vi "Path Flatness SLM.vi"() -> (8 "flatness path":path)   [LabVIEW 2014]
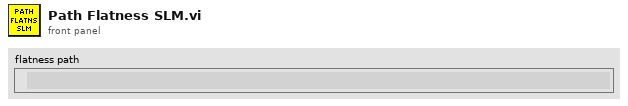
[diagram p1: front panel]
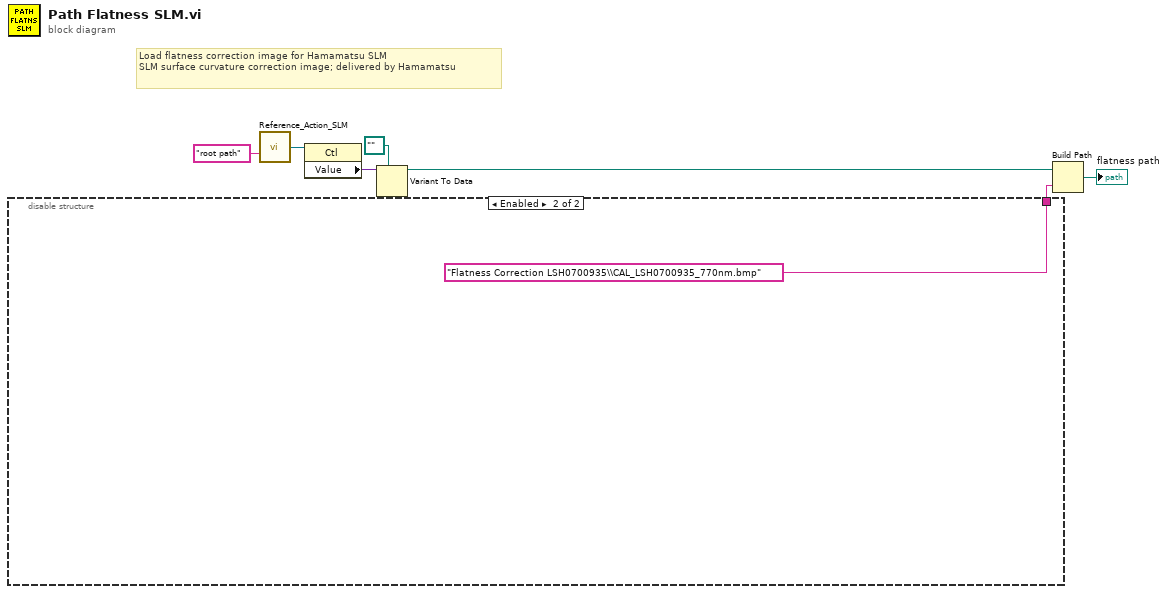
[diagram p0: block diagram]
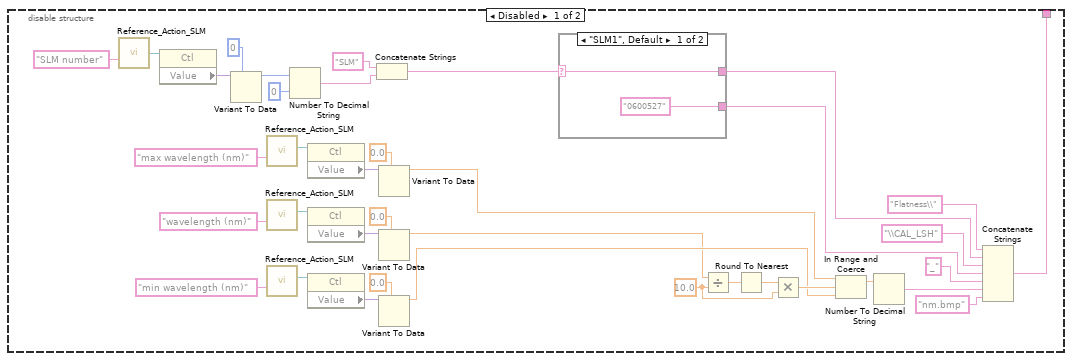
[diagram p2: hidden frame]
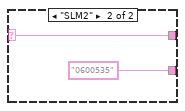
[diagram p3: hidden frame]
diagram:
  # "Load flatness correction image for Hamamatsu SLM\nSLM surface curvature correction image; delivered by Hamamatsu"
  n1 = disable-structure shown="Enabled" {
    disable-tunnel: [w17 "Flatness Correction LSH0700935\\CAL_LSH0700935_770nm.bmp"] -> w2
    frame Disabled {
      w24 = 10.0 ("y")
      n2 = call "Reference_Action_SLM.vi"("Control Name"="SLM number") -> ("Ref OUT"=w13:refnum<vi>)  [unwired: 12 in, 2 out]
      n3 = property class="Ctl"(reference=w13) -> ("Value"=w14:variant)  [unwired: 1 in, 2 out]
      n4 = Variant To Data(type=0, Variant=w14) -> (data=w10:i32)  [unwired: 1 in, 1 out]
      n5 = call "Reference_Action_SLM.vi"("Control Name"="max wavelength (nm)") -> ("Ref OUT"=w43:refnum<vi>)  [unwired: 12 in, 2 out]
      n6 = call "Reference_Action_SLM.vi"("Control Name"="wavelength (nm)") -> ("Ref OUT"=w39:refnum<vi>)  [unwired: 12 in, 2 out]
      n7 = call "Reference_Action_SLM.vi"("Control Name"="min wavelength (nm)") -> ("Ref OUT"=w35:refnum<vi>)  [unwired: 12 in, 2 out]
      n8 = Number To Decimal String(number=w10, width (-)=i16 0) -> (decimal integer string=w8:string)
      n9 = property class="Ctl"(reference=w43) -> ("Value"=w44:variant)  [unwired: 1 in, 2 out]
      n10 = property class="Ctl"(reference=w39) -> ("Value"=w40:variant)  [unwired: 1 in, 2 out]
      n11 = property class="Ctl"(reference=w35) -> ("Value"=w36:variant)  [unwired: 1 in, 2 out]
      n12 = Concatenate Strings("SLM" ("name or relative path"), w8) -> (w15:string)
      n13 = Variant To Data(type=0.0, Variant=w44) -> (data=w20:dbl)  [unwired: 1 in, 1 out]
      n14 = Variant To Data(type=0.0, Variant=w40) -> (data=w21:dbl)  [unwired: 1 in, 1 out]
      n15 = Variant To Data(type=0.0, Variant=w36) -> (data=w22:dbl)  [unwired: 1 in, 1 out]
      n16 = case shown="\"SLM1\", Default" w15 {
        selector: w15 -> [w46 w48]
        tunnel: [w46 w48] -> w18
        tunnel: ["0600527" ("string") "0600535" ("string")] -> w19
        frame "SLM1", Default {
        }
        frame "SLM2" {
        }
      }
      n17 = Divide(x=w21, y=w24) -> (x/y=w26:dbl)
      n18 = Round To Nearest(number=w26) -> (nearest integer value=w25:dbl)
      n19 = Multiply(x=w25, y=w24) -> (x*y=w23:dbl)
      n20 = In Range and Coerce(upper limit=w20, x=w23, lower limit=w22) -> (coerced(x)=w28:dbl)  [unwired: 1 out]
      n21 = Number To Decimal String(number=w28) -> (decimal integer string=w29:string)  [unwired: 1 out]
      n22 = Concatenate Strings("Flatness\\", w18, "\\CAL_LSH", w19, "_" ("string"), w29, "nm.bmp") -> (w17:string)
    }
    frame Enabled {
    }
  }
  n23 = call "Reference_Action_SLM.vi"("Control Name"="root path") -> ("Ref OUT"=w6:refnum<vi>)  [unwired: 12 in, 2 out]
  n24 = property class="Ctl"(reference=w6) -> ("Value"=w5:variant)  [unwired: 1 in, 2 out]
  n25 = Variant To Data(type=path "" ("Path"), Variant=w5) -> (data=w3:path)  [unwired: 1 in, 1 out]
  n26 = Build Path(base path=w3, name or relative path=w2) -> (appended path=→"flatness path":path)
